vi "If_Time_arguments.vi"(0 "seconds since 1Jan1904":dbl, 1 "String Value":string) -> (2 "Error Comments":string, 3 "Time Between?":bool, 4 "Execute Row?":bool)   [LabVIEW 2010]
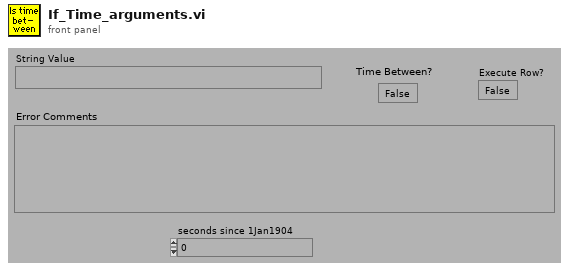
[diagram p1: front panel]
types:
  T1 = cluster{"second":i32, "minute":i32, "hour":i32, "day of month":i32, "month":i32, "year":i32, "day of week":i32, "day of year":i32, "is DST":i32}
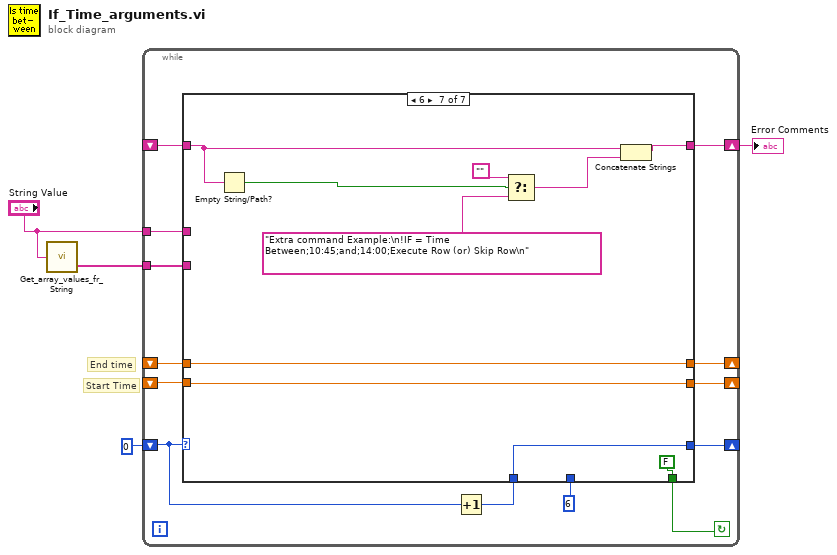
[diagram p0: block diagram]
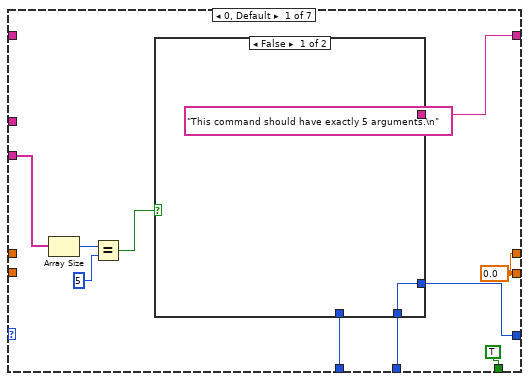
[diagram p2: hidden frame]
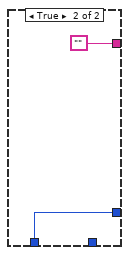
[diagram p3: hidden frame]
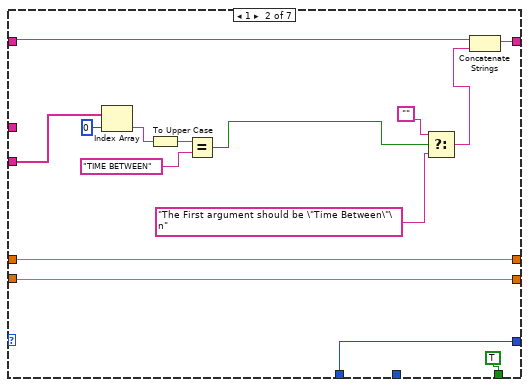
[diagram p4: hidden frame]
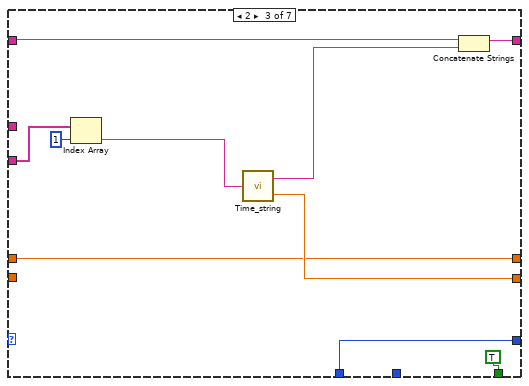
[diagram p5: hidden frame]
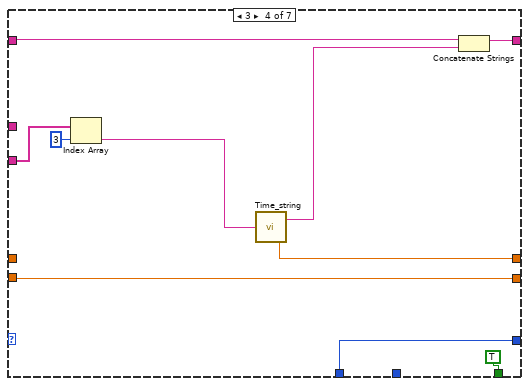
[diagram p6: hidden frame]
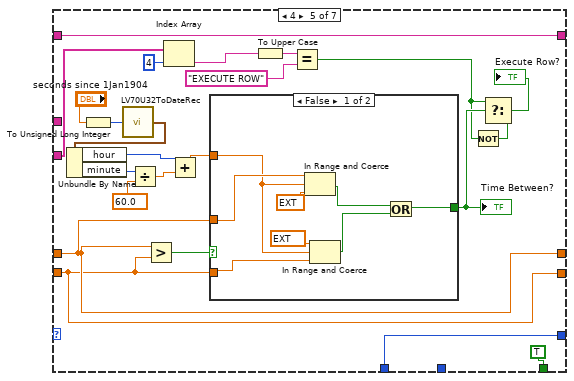
[diagram p7: hidden frame]
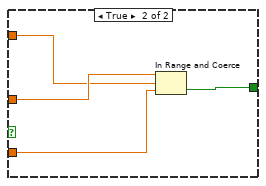
[diagram p8: hidden frame]
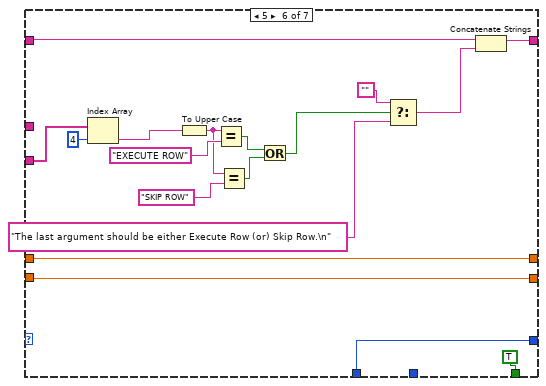
[diagram p9: hidden frame]
diagram:
  # "Start Time"
  # "End time"
  n1 = call "Get_array_values_fr_String.vi"("String Value"="String Value") -> ("String array"=w3:string[])  [unwired: 1 out]
  n2 = while {
    shift-left: _ -> [w5]
    shift-right: [w6] -> _
    tunnel: "String Value" -> [w7]
    shift-left: _ -> [w8]
    shift-right: [w9] -> _
    shift-left: _ -> [w11]
    shift-right: [w12] -> w2
    tunnel: w3 -> [w17]
    shift-left: 0 -> [w16]
    shift-right: [w14] -> _
    stop <- w13 continue-if-true
    n3 = Increment(x=w16) -> (x+1=w15:i32)
    n4 = case shown="6" w16 {
      tunnel: w17 -> [w22 w38 w50 w60 w74 w114 _]
      tunnel: w15 -> [w25 w43 w55 w65 w89 w118 w122]
      tunnel: [w26 w43 w55 w65 w89 w118 w122] -> w14
      tunnel: [TRUE TRUE TRUE TRUE TRUE TRUE FALSE] -> w13
      tunnel: [w27 w40 w52 w62 w87 w115 w124] -> w12
      tunnel: w11 -> [_ w41 w53 w63 w87 w116 w126]
      tunnel: 6 ("t") -> [w23 _ _ _ _ _ _]
      tunnel: [w18 w33 w48 w58 w79 w113 w123] -> w9
      tunnel: w8 -> [_ w33 _ w58 w79 w113 w123]
      tunnel: w7 -> [_ _ _ _ _ _ _]
      tunnel: [w18 w32 w47 w57 w80 w112 w120] -> w6
      tunnel: w5 -> [_ w32 w47 _ w80 w112 w120]
      frame 0, Default {
        w18 = 0.0
        n5 = Array Size(array=w22) -> (size(s)=w21:i32)
        n6 = Equal?(x=w21, y=5) -> (x = y?=w19:bool)
        n7 = case shown="False" w19 {
          tunnel: ["This command should have exactly 5 arguments.\n" ""] -> w27
          tunnel: [w28 w30] -> w26
          tunnel: w25 -> [_ w30]
          tunnel: w23 -> [w28 _]
          frame False {
          }
          frame True {
          }
        }
      }
      frame 1 {
        n8 = Index Array(array=w38, index=0 ("Index")) -> (element=w37:string)
        n9 = To Upper Case(1:w37) -> (0:w36:string)
        n10 = Equal?(x=w36, y="TIME BETWEEN") -> (x = y?=w34:bool)
        n11 = Select(t="", s=w34, f="The First argument should be \"Time Between\"\n" ("Format String")) -> (s? t:f=w39:string)
        n12 = Concatenate Strings(w41, w39) -> (w40:string)
      }
      frame 2 {
        n13 = Index Array(array=w50, index=1 ("Index")) -> (element=w49:string)
        n14 = call "Time_string.vi"("Input String"=w49) -> ("Error String"=w51:string, "24 Hour decimal"=w48:dbl)
        n15 = Concatenate Strings(w53, w51) -> (w52:string)
      }
      frame 3 {
        n16 = Index Array(array=w60, index=3 ("Index")) -> (element=w59:string)
        n17 = call "Time_string.vi"("Input String"=w59) -> ("Error String"=w61:string, "24 Hour decimal"=w57:dbl)
        n18 = Concatenate Strings(w63, w61) -> (w62:string)
      }
      frame 4 {
        n19 = To Unsigned Long Integer(number="seconds since 1Jan1904") -> (unsigned 32bit integer=w67:u32)
        n20 = call <vilib>:"LV70U32ToDateRec.vi"("Time"=w67) -> ("date time rec"=w69:T1)
        n21 = Unbundle By Name(w69) -> ("hour"=w84:i32, "minute"=w86:i32)
        n22 = Divide(x=w86, y=60.0) -> (x/y=w83:dbl)
        n23 = Greater?(x=w80, y=w79) -> (0:w82:bool)
        n24 = Index Array(array=w74, index=4 ("Index")) -> (element=w76:string)
        n25 = Add(x=w84, y=w83) -> (x+y=w81:dbl)
        n26 = case shown="False" w82 {
          tunnel: w80 -> [w97 w101]
          tunnel: w79 -> [w94 w98]
          tunnel: w81 -> [w95 w100]
          tunnel: [w90 w99] -> w73
          frame False {
            (unwired) 0.0
            n27 = In Range and Coerce(upper limit=w97, x=w95, lower limit=ext 0.0 ("lo")) -> (In Range?=w91:bool)  [unwired: 1 out]
            n28 = In Range and Coerce(upper limit=ext 24.0 ("hi"), x=w95, lower limit=w94) -> (In Range?=w92:bool)  [unwired: 1 out]
            n29 = Or(x=w91, y=w92) -> (x .or. y?=w90:bool)
          }
          frame True {
            n30 = In Range and Coerce(upper limit=w101, x=w100, lower limit=w98) -> (In Range?=w99:bool)  [unwired: 1 out]
          }
        }
        "Time Between?" <- w73
        n31 = To Upper Case(1:w76) -> (0:w75:string)
        n32 = Equal?(x=w75, y="EXECUTE ROW") -> (x = y?=w71:bool)
        n33 = Not(x=w71) -> (.not. x?=w70:bool)
        n34 = Select(t=w71, s=w73, f=w70) -> (s? t:f=→"Execute Row?":bool)
      }
      frame 5 {
        n35 = Index Array(array=w114, index=4 ("Index")) -> (element=w110:string)
        n36 = To Upper Case(1:w110) -> (0:w108:string)
        n37 = Equal?(x=w108, y="EXECUTE ROW") -> (x = y?=w106:bool)
        n38 = Equal?(x=w108, y="SKIP ROW") -> (x = y?=w107:bool)
        n39 = Or(x=w106, y=w107) -> (x .or. y?=w104:bool)
        n40 = Select(t="", s=w104, f="The last argument should be either Execute Row (or) Skip Row.\n" ("y")) -> (s? t:f=w105:string)
        n41 = Concatenate Strings(w116, w105) -> (w115:string)
      }
      frame 6 {
        n42 = Empty String/Path?(string/path=w126) -> (empty?=w129:bool)
        n43 = Select(t="", s=w129, f="Extra command Example:\n!IF = Time Between;10:45;and;14:00;Execute Row (or) Skip Row\n") -> (s? t:f=w127:string)
        n44 = Concatenate Strings(w126, w127) -> (w124:string)
      }
    }
  }
  "Error Comments" <- w2
